vi "RIGOL DP800 Series Output DC Volts.vi"() -> ()   [LabVIEW 2020, in "Library Instrument & Equipement.lvlib" / "Library Power_Supply.lvlib" / "RIGOL DP800 Series.lvlib"]
doc: "This example shows how to configure the instrument's output voltage level, over current protection, and over voltage protection. The actual voltage level and actual current level are returned as well as whether over voltage protection (OVP) or over current protection (OCP) has been tripped."
uses:
  RIGOL DP800 Series.lvlib
  Channels.ctl
panel:
  in  "Enable OCP (T: Enable)":bool=TRUE caption="Enable OVP (T: Enable)"
  in  "Current Level (0.0 V)":dbl caption="Voltage Level (0.0 V)" format="%.2f"
  in  "Output Voltage":bool=TRUE caption="Enable OVP (T: Enable)"
  in  "Bouton Annuler":bool
  in  "Bouton Open":bool
  in  "Channel (0: 30V Channel)":T1 caption="Channel (0: +6V)" items=["30V/3A Channel", "30V/3A Channel", "5V/3A Channel"]
  in  "Enable OVP (T: Enable)":bool=TRUE
  in  "Voltage Limit (0V)":dbl format="%.2f"
  in  "Voltage Level (0.0 V)":dbl format="%.2f"
  in  "Current Limit (0A)":dbl format="%.2f"
  in  "VISA resource name":refnum<visa-resource-name>
  # "Over Voltage Protection"
  # "Over Current Protection"
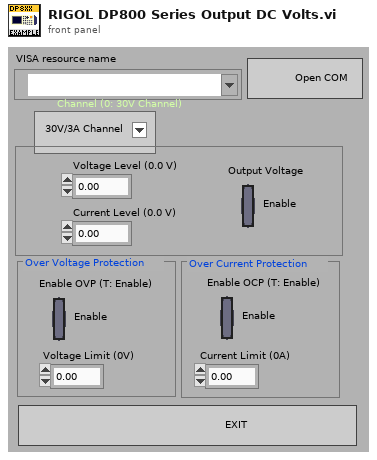
[diagram p1: front panel]
types:
  T1 = typedef "Library Instrument & Equipement.lvlib/Library Power_Supply.lvlib/RIGOL DP800 Series.lvlib/Channels.ctl" = i32
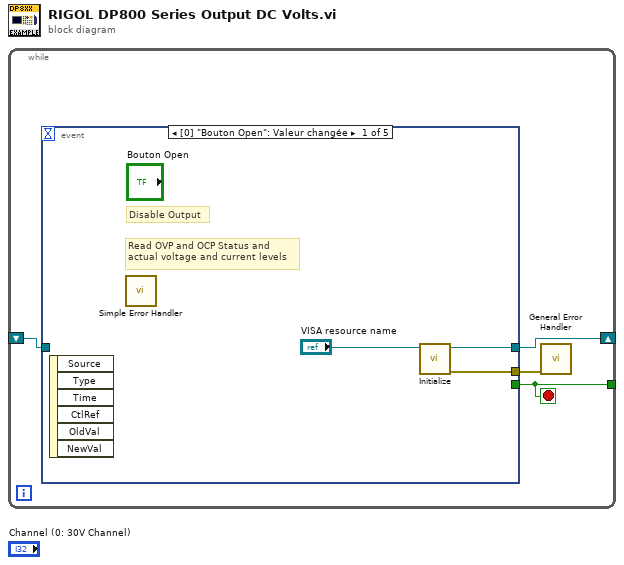
[diagram p0: block diagram]
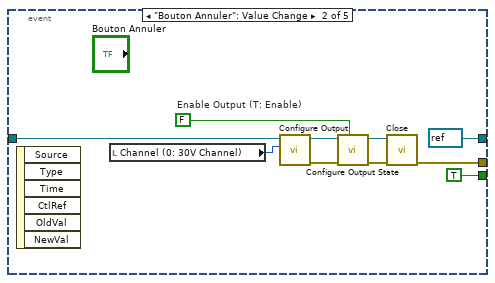
[diagram p2: hidden frame]
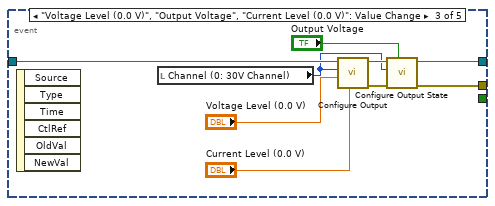
[diagram p3: hidden frame]
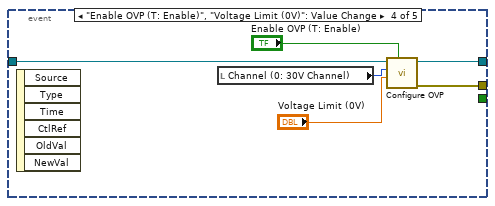
[diagram p4: hidden frame]
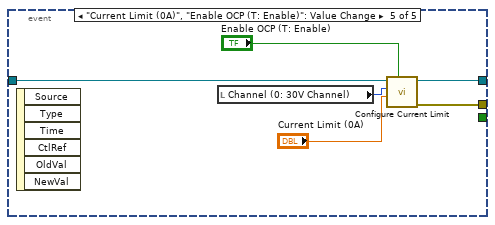
[diagram p5: hidden frame]
diagram:
  n1 = while {
    tunnel: [w4] -> _
    shift-right: [w3] -> _
    shift-left: _ -> [w2]
    stop <- w4 stop-if-true
    n2 = event shown="[0] \"Bouton Open\": Valeur changée" {
      selector: _ -> [_ _ _ _ _]
      dyn-events: _ -> [_ _ _ _ _]
      timeout: _ -> [_ _ _ _ _]
      tunnel: [_ TRUE _ _ _] -> w4
      tunnel: [w6 refnum<visa-resource-name> refnum ("VISA resource name out") w20 w27 w34] -> w3
      tunnel: w2 -> [_ w14 w26 w29 w36]
      tunnel: [w5 w15 w22 w28 w37] -> w1
      event "Bouton Open": Value Change {
        # "Disable Output"
        # "Read OVP and OCP Status and\nactual voltage and current levels"
        n3 = event-data() -> ()  [unwired: 1 in, 6 out]
        n4 = call <vilib>:"Simple Error Handler.vi"() -> ()  [unwired: 2 in, 8 out]
        n5 = call "Initialize.vi"("VISA resource name"="VISA resource name") -> ("error out"=w5:errorcluster, "VISA resource name out"=w6:refnum<visa-resource-name>)  [unwired: 9 in]
      }
      event "Bouton Annuler": Value Change {
        w10 = FALSE  # Enable Output (T: Enable)
        n6 = event-data() -> ()  [unwired: 1 in, 6 out]
        n7 = local read "Channel (0: 30V Channel)"() -> (w16:T1)
        n8 = call "Configure Output.vi"("Channel (0: 30V Channel)"=w16, "VISA resource name"=w14) -> ("error out"=w12:errorcluster, "VISA resource name out"=w9:refnum<visa-resource-name>)  [unwired: 8 in]
        n9 = call "Configure Output State.vi"("Enable Output (T: Enable)"=w10, "error in (no error)"=w12, "VISA resource name"=w9) -> ("error out"=w11:errorcluster, "VISA resource name out"=w8:refnum<visa-resource-name>)  [unwired: 7 in]
        n10 = call "Close.vi"("error in (no error)"=w11, "VISA resource name"=w8) -> ("error out"=w15:errorcluster)  [unwired: 9 in]
      }
      event "Voltage Level (0.0 V)", "Output Voltage", "Current Level (0.0 V)": Value Change {
        n11 = event-data() -> ()  [unwired: 1 in, 6 out]
        n12 = local read "Channel (0: 30V Channel)"() -> (w18:T1)
        n13 = call "Configure Output.vi"("Curent Level (0.0 V)"="Current Level (0.0 V)", "Voltage Level (0.0 V)"="Voltage Level (0.0 V)", "Channel (0: 30V Channel)"=w18, "VISA resource name"=w26) -> ("error out"=w23:errorcluster, "VISA resource name out"=w21:refnum<visa-resource-name>)  [unwired: 6 in]
        n14 = call "Configure Output State.vi"("Enable Output (T: Enable)"="Output Voltage", "error in (no error)"=w23, "Channel (0: 30V Channel)"=w18, "VISA resource name"=w21) -> ("error out"=w22:errorcluster, "VISA resource name out"=w20:refnum<visa-resource-name>)  [unwired: 6 in]
      }
      event "Enable OVP (T: Enable)", "Voltage Limit (0V)": Value Change {
        n15 = event-data() -> ()  [unwired: 1 in, 6 out]
        n16 = local read "Channel (0: 30V Channel)"() -> (w30:T1)
        n17 = call "Configure OVP.vi"("Enable OVP (T: Enable)"="Enable OVP (T: Enable)", "Voltage Limit (6.5 V)"="Voltage Limit (0V)", "Channel (0: 30V Channel)"=w30, "VISA resource name"=w29) -> ("error out"=w28:errorcluster, "VISA resource name out"=w27:refnum<visa-resource-name>)  [unwired: 6 in]
      }
      event "Current Limit (0A)", "Enable OCP (T: Enable)": Value Change {
        n18 = event-data() -> ()  [unwired: 1 in, 6 out]
        n19 = local read "Channel (0: 30V Channel)"() -> (w35:T1)
        n20 = call "Configure Current Limit.vi"("Enable OCP (T: Enable)"="Enable OCP (T: Enable)", "Current Limit (5.0 A)"="Current Limit (0A)", "Channel (0: 30V Channel)"=w35, "VISA resource name"=w36) -> ("error out"=w37:errorcluster, "VISA resource name out"=w34:refnum<visa-resource-name>)  [unwired: 6 in]
      }
    }
    n21 = call <vilib>:"General Error Handler.vi"("error in (no error)"=w1) -> ()  [unwired: 10 in, 5 out]
  }
